vi "SignalSenderLoop.111.vi"(8 "error in (no error)":errorcluster, 10 "111":T1, 11 "SignalSenderLoop":refnum<class "SignalSenderLoop.lvclass">) -> (0 "error out":errorcluster, 3 "SignalSenderLoop out":refnum<class "SignalSenderLoop.lvclass">)   [LabVIEW 2020, in "SignalSenderLoop.lvclass"]
doc: "---------------------------------------------------------------\nJKI State Machine Objects™\nhttp://jki.net/state-machine-objects/\nCopyright (C) 2005-2015, JKI <info@jki.net>\nALL RIGHTS RESERVEDJKI State Machine Objects (SMO) 1.0.0.4\nJKI - JKI\nCopyright (c) 2015, JKI"
uses:
  SignalSenderLoop.lvclass
  Typedefs/PrivateEvents--SignalSenderLoop.111.ctl
  SignalSenderLoop.lvclass/SignalSenderLoop.ctl
panel:
  # "For instructions on how to use the JKI State Machine Objects, examples and video tutorials, visit:\nhttp://jki.net/state-machine-objects/\n\nJKI State Machine Objects™\nhttp://jki.net/state-machine-objects/\nCopyright (C) 2005-2015, JKI <info@jki.net>\nALL RIGHTS RESERVED"
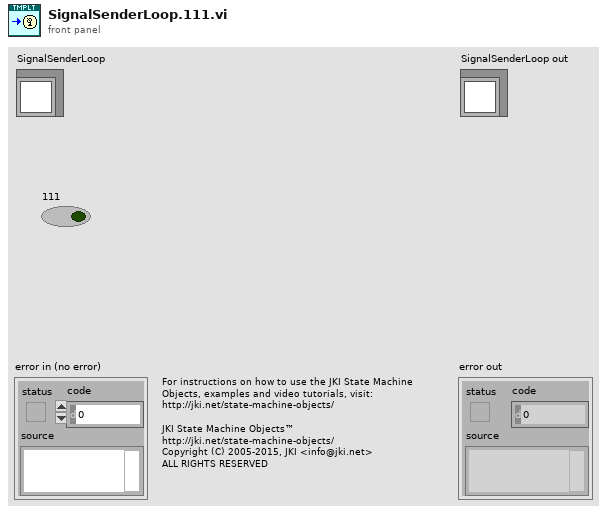
[diagram p1: front panel]
types:
  T1 = typedef "SignalSenderLoop.lvclass/PrivateEvents--SignalSenderLoop.111.ctl" = bool
  T2 = typedef "SignalSenderLoop.lvclass/PrivateData--Ref.ctl" = refnum<data-value>
  T3 = typedef "SignalSenderLoop.lvclass/PrivateData--Cluster.ctl" = cluster{"Public Events":T4, "Setpoint":T5, "Private Events":T6, "信号轮询发送设置":T7}
  T4 = typedef "SignalSenderLoop.lvclass/PublicEvents--Cluster.ctl" = cluster{"Setpoint Changed":refnum<user-event>, "Value Changed":refnum<user-event>}
  T5 = typedef "SignalSenderLoop.lvclass/Data.ctl" = dbl
  T6 = typedef "SignalSenderLoop.lvclass/PrivateEvents--Cluster.ctl" = cluster{"AsyncMethod":refnum<user-event>, "111":refnum<user-event>}
  T7 = typedef "SignalSenderLoop.lvclass/信号轮询发送设置.ctl" = cluster{"XNET SignalFrameArry":T8[]}
  T8 = typedef "SignalFrameSet.ctl" = cluster{"Port_No.":refnum<k21>, "XNETSignals":refnum<k21>[], "计数Count":bool, "校验CheckSum":bool}
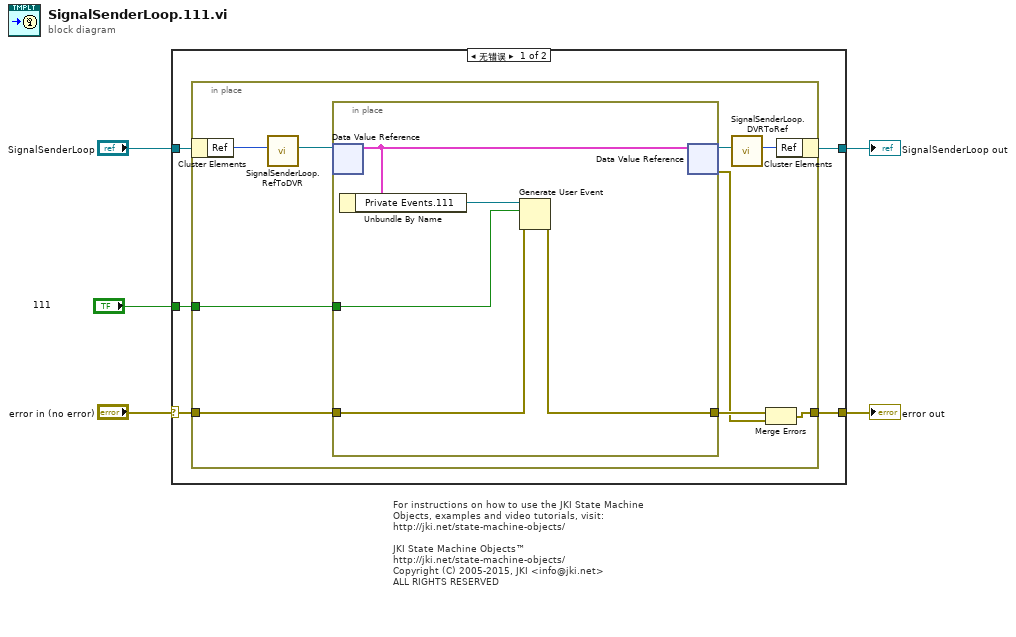
[diagram p0: block diagram]
diagram:
  # "For instructions on how to use the JKI State Machine Objects, examples and video tutorials, visit:\nhttp://jki.net/state-machine-objects/\n\nJKI State Machine Objects™\nhttp://jki.net/state-machine-objects/\nCopyright (C) 2005-2015, JKI <info@jki.net>\nALL RIGHTS RESERVED"
  n1 = case shown="无错误" "error in (no error)" {
    selector: "error in (no error)" -> [w8 w26]
    tunnel: [w7 w26] -> w4
    tunnel: [w9 w25] -> w5
    tunnel: "SignalSenderLoop" -> [w10 w25]
    tunnel: "111" -> [w6 _]
    frame No Error {
      n2 = in-place {
        in-place-border: w8 -> [w19]
        in-place-border: [w16] -> w7
        in-place-border: w6 -> [w13]
        n3 = in-place-cluster #1(w10) -> ("Ref"=w15:u32)
        n4 = call "SignalSenderLoop.RefToDVR.vi"("Ref"=w15) -> ("Ref"=w12:T2)  [unwired: 10 in]
        n5 = in-place {
          in-place-border: w19 -> [w22]
          in-place-border: [w21] -> w18
          in-place-border: w13 -> [w20]
          n6 = in-place-dvr #2(w12) -> (w24:T3)  [unwired: 1 out]
          n7 = Unbundle By Name(w24) -> ("Private Events.111"=w23:refnum<user-event>)
          n8 = Generate User Event(user event=w23, event data cluster=w20, error in=w22) -> (error out=w21:errorcluster)  [unwired: 1 in, 1 out]
          n9 = in-place-dvr #2(w24) -> (w14:T2, w17:errorcluster)
        }
        n10 = call "SignalSenderLoop.DVRToRef.vi"("Ref"=w14) -> ("Ref"=w11:u32)  [unwired: 10 in]
        n11 = Merge Errors(w18, w17) -> (w16:errorcluster)
        n12 = in-place-cluster #1("Ref"=w11) -> (w9:refnum<class "SignalSenderLoop.lvclass">)
      }
    }
    frame Error {
    }
  }
  "error out" <- w4
  "SignalSenderLoop out" <- w5
